vi "AtualizaPainel.vi"(0 "VI in":refnum<vi>, 2 "Init":bool, 4 "ParamsIn":variant) -> (16 "ParamsOut":variant)   [LabVIEW 2017]
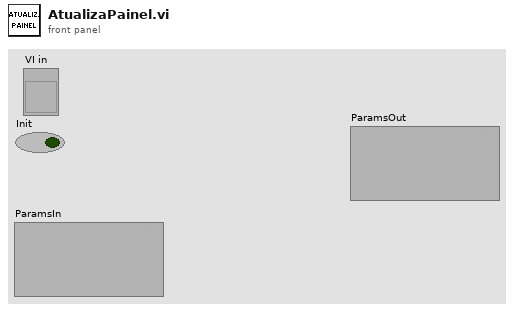
[diagram p1: front panel]
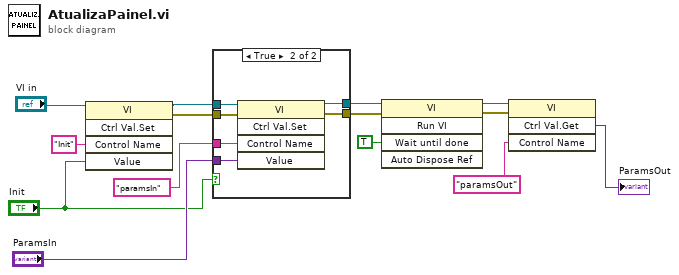
[diagram p0: block diagram]
diagram:
  n1 = invoke class="VI" method="Ctrl Val.Set"(reference="VI in", "Control Name"="Init", "Value"="Init") -> (reference out=w7:refnum<vi>, error out=w6:errorcluster)  [unwired: 2 in, 3 out]
  n2 = case shown="True" "Init" {
    tunnel: w7 -> [w16 w22]
    tunnel: w6 -> [w15 w21]
    tunnel: "ParamsIn" -> [_ w20]
    tunnel: [w16 w19] -> w4
    tunnel: [w15 w18] -> w3
    tunnel: "paramsIn" ("Control Name") -> [_ w17]
    frame False {
    }
    frame True {
      n3 = invoke class="VI" method="Ctrl Val.Set"(reference=w22, error in=w21, "Control Name"=w17, "Value"=w20) -> (reference out=w19:refnum<vi>, error out=w18:errorcluster)  [unwired: 1 in, 3 out]
    }
  }
  n4 = invoke class="VI" method="Run VI"(reference=w4, error in=w3, "Wait until done"=TRUE ("Wait Until Done")) -> (reference out=w12:refnum<vi>, error out=w13:errorcluster)  [unwired: 2 in, 3 out]
  n5 = invoke class="VI" method="Ctrl Val.Get"(reference=w12, error in=w13, "Control Name"="paramsOut") -> ("Get Control Value Variant"=→"ParamsOut":variant)  [unwired: 1 in, 3 out]
